vi "PIEZO_monitor_Position.vi"(3 "handle":i32, 4 "error in":errorcluster, 5 "Zposition setpoint":dbl) -> (1 "error out":errorcluster, 2 "Z":dbl)   [LabVIEW 2015]
uses:
  <userlib>/Madlib.dll
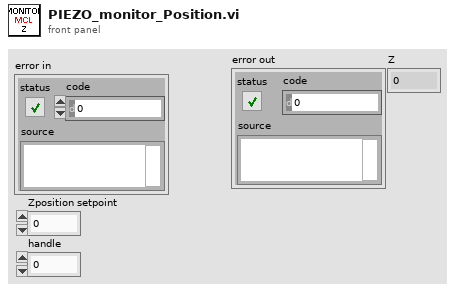
[diagram p1: front panel]
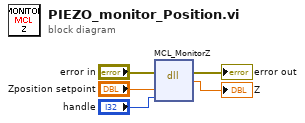
[diagram p0: block diagram]
diagram:
  n1 = dll-call lib="C:/Program Files/National Instruments/LabVIEW 2015/user.lib/Madlib.dll" fn="MCL_MonitorZ"(error in="error in", "setpoint"="Zposition setpoint", "handle"="handle") -> (error out=→"error out":errorcluster, "Z"=→"Z":dbl)  [unwired: 4 in, 1 out]
